vi "Read Name.vi"(11 "Network Stream in":refnum<class "Network Stream.lvclass">) -> (2 "Name":string)   [LabVIEW 2020, in "Network Stream.lvclass"]
doc: "Returns the name for this network stream."
uses:
  Network Stream.lvclass
  Network Stream.lvclass/Network Stream.ctl
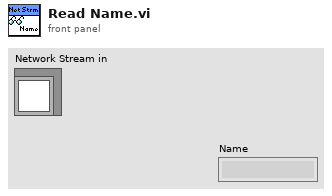
[diagram p1: front panel]
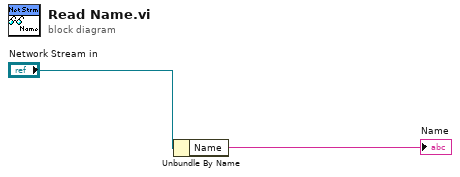
[diagram p0: block diagram]
diagram:
  n1 = Unbundle By Name("Network Stream in") -> ("Name"=→"Name":string)
